vi "DriveTeleOp.vi"(10 "Axes":dbl[](array[numeric]), 11 "Robot":T1) -> ()   [LabVIEW 2015]
uses:
  Robot Type Def.ctl
  Framework/Robot Global Data.vi
  Drive/Implementation/RobotDriveGlobal.vi
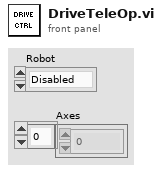
[diagram p1: front panel]
types:
  T1 = typedef "Robot Type Def.ctl" = enum32{"Disabled", "Ghost", "Casper", "Lofty", "Board", "RaceRobot", "Casper 2.0", "Excalibot 2.0"}
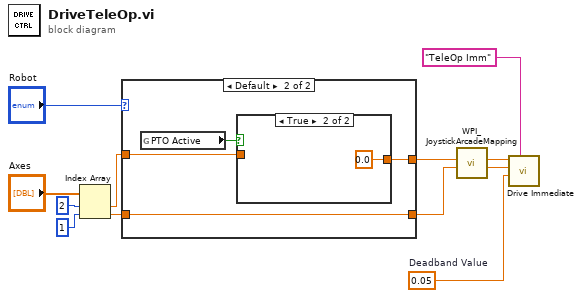
[diagram p0: block diagram]
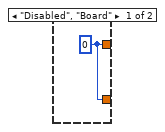
[diagram p2: hidden frame]
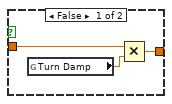
[diagram p3: hidden frame]
diagram:
  w8 = 0.05  # Deadband Value
  n1 = Index Array(array="Axes", index #1=2 ("index"), index #2=1 ("index")) -> (element #1=w6:dbl, element #2=w10:dbl)
  n2 = case shown="Default" "Robot" {
    tunnel: w6 -> [_ w15]
    tunnel: [w13 w16] -> w7
    tunnel: [w13 w14] -> w9
    tunnel: w10 -> [_ w14]
    frame "Disabled", "Board" {
      w13 = 0
    }
    frame Default {
      n3 = global read "Robot Global Data.vi" "PTO Active"() -> (w17:bool)
      n4 = case shown="True" w17 {
        tunnel: w15 -> [w20 _]
        tunnel: [w19 0.0] -> w16
        frame False {
          n5 = global read "RobotDriveGlobal.vi" "Turn Damp"() -> (w18:dbl)
          n6 = Multiply(x=w20, y=w18) -> (x*y=w19:dbl)
        }
        frame True {
        }
      }
    }
  }
  n7 = call <vilib>:"WPI_JoystickArcadeMapping.vi"("Y axis value"=w9, "X axis value"=w7) -> ("Right Motor Value"=w3:dbl, "Left Motor Value"=w2:dbl)  [unwired: 8 in]
  n8 = call "Drive Immediate.vi"("Description"="TeleOp Imm", "Deadband Value"=w8, "Right Setpoint"=w3, "Left Setpoint"=w2) -> ()  [unwired: 7 in, 1 out]
